vi "Measurement Display.vi"(5 "Boolean":bool, 7 "Frequency In":dbl, 8 "Tension In":dbl, 9 "Wire Length In":dbl, 10 "Linear Density In":dbl, 11 "dT In":dbl) -> (0 "Wire Length Out":dbl, 1 "dT Out":dbl, 2 "Tension Out":dbl, 3 "Frequency Out":dbl, 4 "Linear Density Out":dbl)   [LabVIEW 2018]
panel:
  # "Inputs"
  # "Outputs"
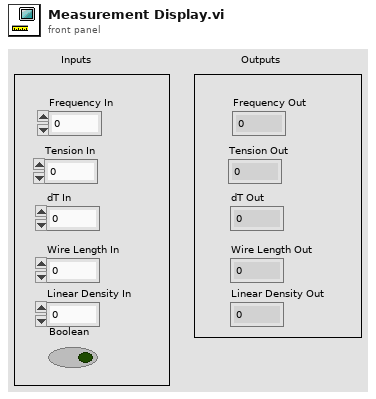
[diagram p1: front panel]
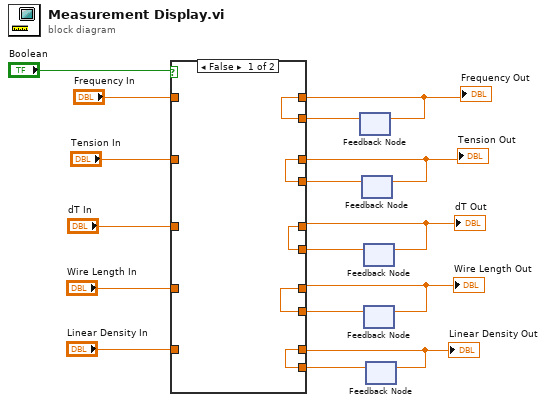
[diagram p0: block diagram]
diagram:
  n1 = feedback #1() -> (w9:dbl)  [unwired: 1 in]
  n2 = feedback #2() -> (w7:dbl)  [unwired: 1 in]
  n3 = feedback #3() -> (w5:dbl)  [unwired: 1 in]
  n4 = feedback #4() -> (w3:dbl)  [unwired: 1 in]
  n5 = feedback #5() -> (w1:dbl)  [unwired: 1 in]
  n6 = case shown="False" "Boolean" {
    tunnel: "Frequency In" -> [_ w26]
    tunnel: "Tension In" -> [_ w25]
    tunnel: "dT In" -> [_ w24]
    tunnel: "Wire Length In" -> [_ w23]
    tunnel: "Linear Density In" -> [_ w22]
    tunnel: [w21 w26] -> w10
    tunnel: [w20 w25] -> w8
    tunnel: [w19 w24] -> w6
    tunnel: [w18 w23] -> w4
    tunnel: [w17 w22] -> w2
    tunnel: w9 -> [w21 _]
    tunnel: w7 -> [w20 _]
    tunnel: w5 -> [w19 _]
    tunnel: w3 -> [w18 _]
    tunnel: w1 -> [w17 _]
    frame False {
    }
    frame True {
    }
  }
  "Frequency Out" <- w10
  "Tension Out" <- w8
  "dT Out" <- w6
  "Wire Length Out" <- w4
  "Linear Density Out" <- w2
  n7 = feedback-in #1(w10) -> ()
  n8 = feedback-in #2(w8) -> ()
  n9 = feedback-in #3(w6) -> ()
  n10 = feedback-in #4(w4) -> ()
  n11 = feedback-in #5(w2) -> ()
